vi "PTSequencer.DIM update once.vi"(0 "i ref in":refnum<vi>, 3 "ms timeout (10000)":i32=10000, 5 "error in":errorcluster) -> (14 "i ref out":refnum<vi>, 17 "timed out":bool, 19 "error out":errorcluster)   [LabVIEW 2014, in "PTSequencer.lvlib"]
uses:
  PTSequencer.lvlib
  CSlibraries-extern/DimLVEvent/LVDimInterface/LVDimInterface.lvlib
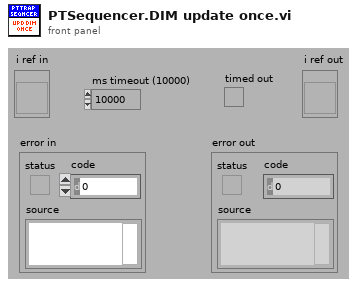
[diagram p1: front panel]
types:
  T1 = typedef "PTSequencer.lvlib/PTSequencer.i attribute.ctl" = cluster{"subsequence":bool, "mode":T2, "i step":i32, "nofLoops":i32, "i loop":i32, "Running":bool, "Paused":bool, "step done":bool, "loop done":bool, "seq done":bool, "DIM IDs":cluster{"step done":i32, "loop done":i32, "seq done":i32, "i step":i32, "i loop":i32}, "use stop conditions":bool, "stop conditions":T3[], "Step List":T5[], "DIM subsriptions":string[], "stop cond indexes":i32[], "step cond indexes":cluster{"step condition IDs":cluster{"step ID":i32, "condition ID":i32}[]}[], "Delay Start Time":timestamp, "status":string, "stopping":bool}
  T2 = typedef "PTSequencer.lvlib/PTSequencer.mode.ctl" = enum16{"single", "loop", "for loop"}
  T3 = typedef "PTSequencer.lvlib/PTSequencer.DIM service condition.ctl" = cluster{"DIM service":string, "descr":string, "nomValue":T4, "actValue":T4, "matched":bool, "DIM Status":cluster{"no link":bool, "quality":i32, "Time Stamp":timestamp}}
  T4 = typedef "CoreDefs.rawDataType.ctl" = i8[]
  T5 = typedef "PTSequencer.lvlib/PTSequencer.step.ctl" = cluster{"description":string, "object parameters":cluster{"object":string, "selector":string, "descriptor":string, "data":T4, "subsequence":bool, "call mode":enum16{"Simple DIM", "Synchronous"}, "data in":T4}, "result action":cluster{"check":bool, "passed":enum16{"Next", "Previous", "Repeat", "Jump"}, "failed":enum16{"Next", "Previous", "Repeat", "Jump"}, "jumpID_passed":i32, "jumpID_failed":i32}, "conditions":T3[], "fulfilled ":bool, "use delay":bool, "delay time (s)":dbl, "ID":i32}
  T6 = cluster{"step condition IDs":cluster{"step ID":i32, "condition ID":i32}[]}[]
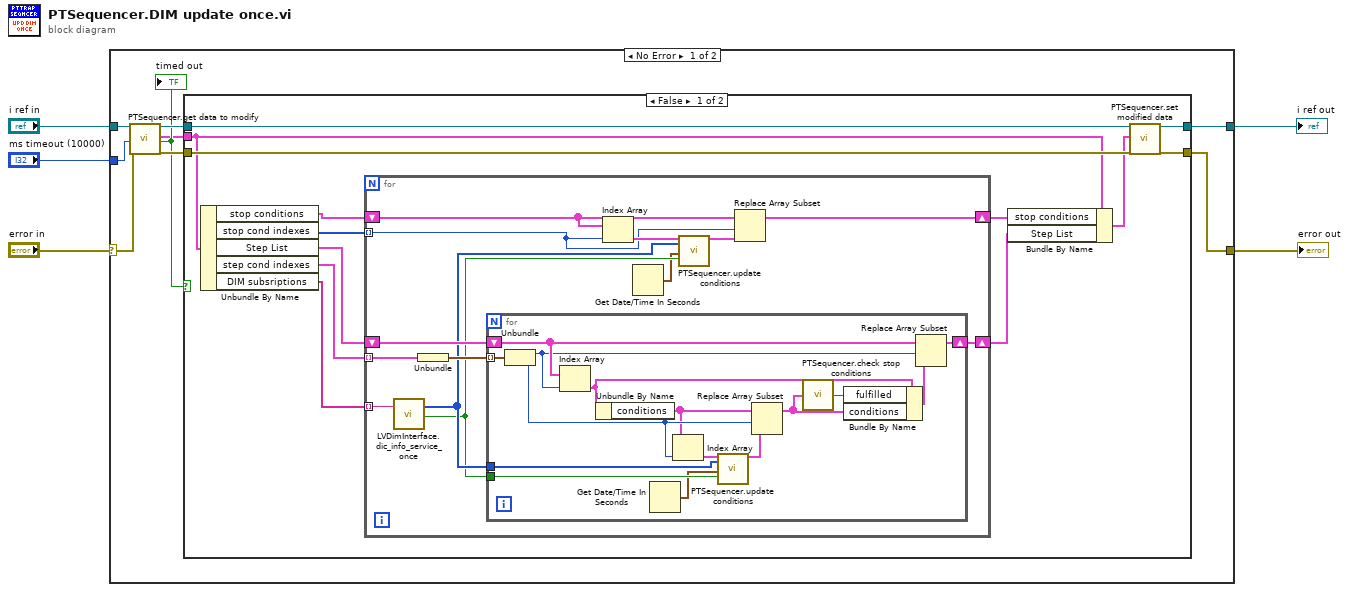
[diagram p0: block diagram]
diagram:
  n1 = case shown="No Error" "error in" {
    selector: "error in" -> [w14 w58]
    tunnel: "i ref in" -> [w11 w59]
    tunnel: [w6 w59] -> w4
    tunnel: [w7 w58] -> w3
    tunnel: "ms timeout (10000)" -> [w8 _]
    frame No Error {
      n2 = call "PTSequencer.get data to modify.vi"("i ref in"=w11, "ms timeout (10000)"=w8, "error in (no error)"=w14) -> ("i ref out"=w12:refnum<vi>, "i attribute"=w9:T1, "timed out"=w10:bool, "error out"=w13:errorcluster)  [unwired: 13 in]
      "timed out" <- w10
      n3 = case shown="False" w10 {
        tunnel: [w15 w57] -> w6
        tunnel: w13 -> [w26 w56]
        tunnel: w12 -> [w27 w57]
        tunnel: w9 -> [w20 _]
        tunnel: [w16 w56] -> w7
        frame False {
          n4 = Unbundle By Name(w20) -> ("stop conditions"=w25:T3[], "stop cond indexes"=w24:i32[], "Step List"=w23:T5[], "step cond indexes"=w22:T6, "DIM subsriptions"=w21:string[])
          n5 = for {
            tunnel: w24 -> [w37] mode=indexing
            tunnel: w22 -> [w36] mode=indexing
            tunnel: w21 -> [w33] mode=indexing
            shift-right: [w28] -> w19
            shift-left: w25 -> [w38]
            shift-right: [w29] -> w18
            shift-left: w23 -> [w34]
            n6 = call "LVDimInterface.dic_info_service_once.vi"("serviceName"=w33) -> ("data"=w32:i8[], "timed out?"=w31:bool)  [unwired: 15 in, 2 out]
            n7 = Unbundle(w36) -> ("step condition IDs"=w35:cluster{"step ID":i32, "condition ID":i32}[])
            n8 = for {
              tunnel: w35 -> [w55] mode=indexing
              shift-right: [w49] -> w29
              shift-left: w34 -> [w53]
              tunnel: w32 -> [w43]
              tunnel: w31 -> [w42]
              n9 = Unbundle(w55) -> ("step ID"=w52:i32, "condition ID"=w54:i32)
              n10 = Index Array(array=w53, index=w52) -> (element=w51:T5)
              n11 = Unbundle By Name(w51) -> ("conditions"=w46:T3[])
              n12 = Get Date/Time In Seconds() -> (seconds since 1Jan1904=w41:timestamp)
              n13 = Index Array(array=w46, index=w54) -> (element=w48:T3)
              n14 = call "PTSequencer.update conditions.vi"("condition in"=w48, "data"=w43, "Time Stamp"=w41, "no link"=w42) -> ("condition out"=w47:T3)  [unwired: 15 in]
              n15 = Replace Array Subset(array=w46, new element=w47, index=w54) -> (w45:T3[])
              n16 = call "PTSequencer.check stop conditions.vi"("conditions"=w45) -> ("fulfilled"=w44:bool)
              n17 = Bundle By Name(cluster=w51, "fulfilled"=w44, "conditions"=w45) -> (w50:T5)
              n18 = Replace Array Subset(array=w53, new element=w50, index=w52) -> (w49:T5[])
            }
            n19 = Index Array(array=w38, index=w37) -> (element=w40:T3)
            n20 = Get Date/Time In Seconds() -> (seconds since 1Jan1904=w30:timestamp)
            n21 = call "PTSequencer.update conditions.vi"("condition in"=w40, "data"=w32, "Time Stamp"=w30, "no link"=w31) -> ("condition out"=w39:T3)  [unwired: 15 in]
            n22 = Replace Array Subset(array=w38, new element=w39, index=w37) -> (w28:T3[])
          }
          n23 = Bundle By Name(cluster=w20, "stop conditions"=w19, "Step List"=w18) -> (w17:T1)
          n24 = call "PTSequencer.set modified data.vi"("i ref in"=w27, "CLASS.i attribute"=w17, "error in (no error)"=w26) -> ("i ref out"=w15:refnum<vi>, "error out"=w16:errorcluster)  [unwired: 15 in]
        }
        frame True {
        }
      }
    }
    frame Error {
    }
  }
  "i ref out" <- w4
  "error out" <- w3
